vi "HeaterAlarmStatusChanged.vi"(7 "ControlQueue":refnum<queue>, 8 "error in (no error)":errorcluster, 9 "HeaterAlarmStatus":bool, 10 "HeaterAlarmStatusChanged":bool, 11 "DAQmxTaksContainer_General in":refnum<class "DAQmxTaksContainer_General.lvclass">) -> (0 "error out":errorcluster, 2 "Alarm":bool, 3 "DAQmxTaksContainer_General out":refnum<class "DAQmxTaksContainer_General.lvclass">)   [LabVIEW 2020, in "DAQmxTaksContainer_General.lvclass"]
uses:
  DAQmxTaksContainer_General.lvclass
  C:/dev/TRANCON/Classes/GeneralFunctionality/GeneralFunctionality.lvclass
  DAQmxTaksContainer_General.lvclass/DAQmxTaksContainer_General.ctl
  dependecies/ControlsVIs/Clusters-def/Standard Command.ctl
  dependecies/ControlsVIs/Clusters-def/SERVER-Commands.ctl
  dependecies/ControlsVIs/Clusters-def/ProtypeCommand-DAQmxReply.ctl
  dependecies/ControlsVIs/Clusters-def/Message types.ctl
  DAQmxTask.lvclass
  Control/Control-Server/Control-Server.lvclass
  Message/Message.lvclass
  GeneralFunctionality/GeneralFunctionality.lvclass
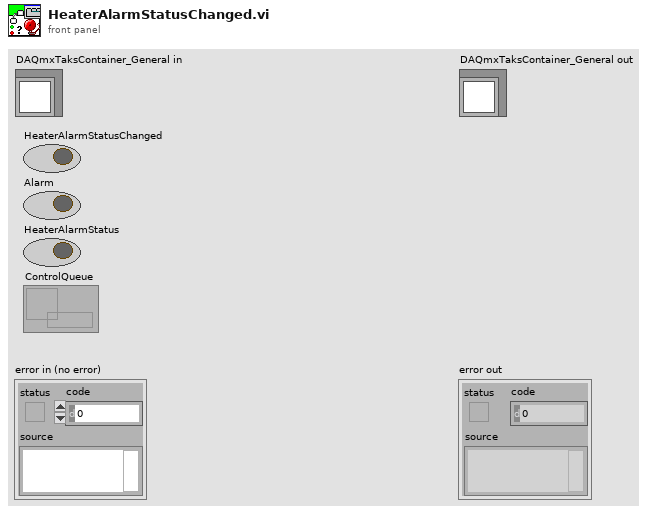
[diagram p1: front panel]
types:
  T1 = typedef "Message types.ctl" = string
  T2 = typedef "ProtypeCommand-DAQmxReply.ctl" = cluster{"On/Off":bool, "error out":errorcluster}
  T3 = typedef "Control-Server.lvclass/SERVER-Commands.ctl" = string
  T4 = typedef "Standard Command.ctl" = cluster{"command":string, "data":variant}
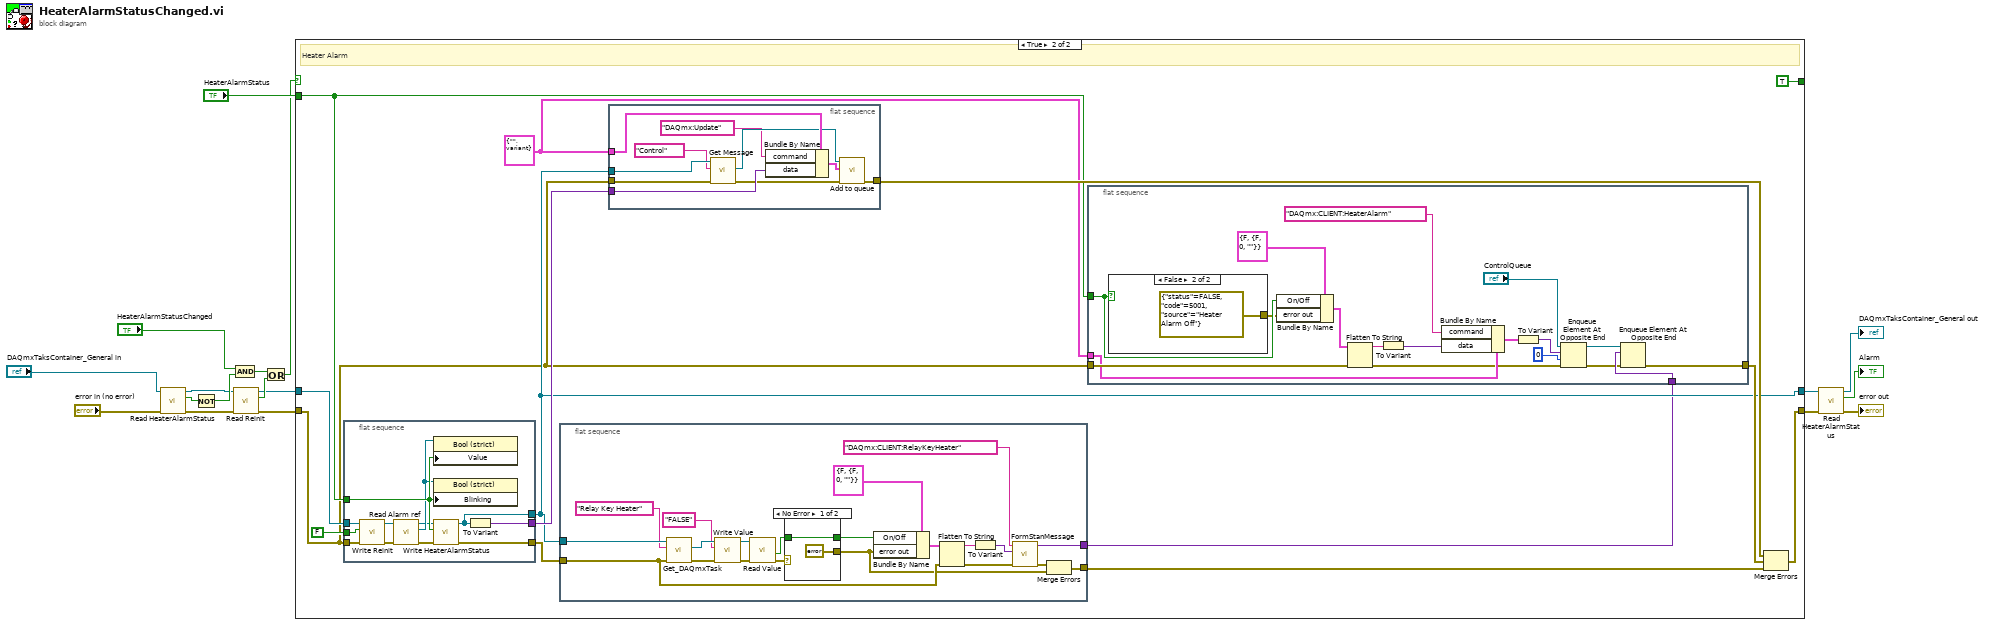
[diagram p0: block diagram]
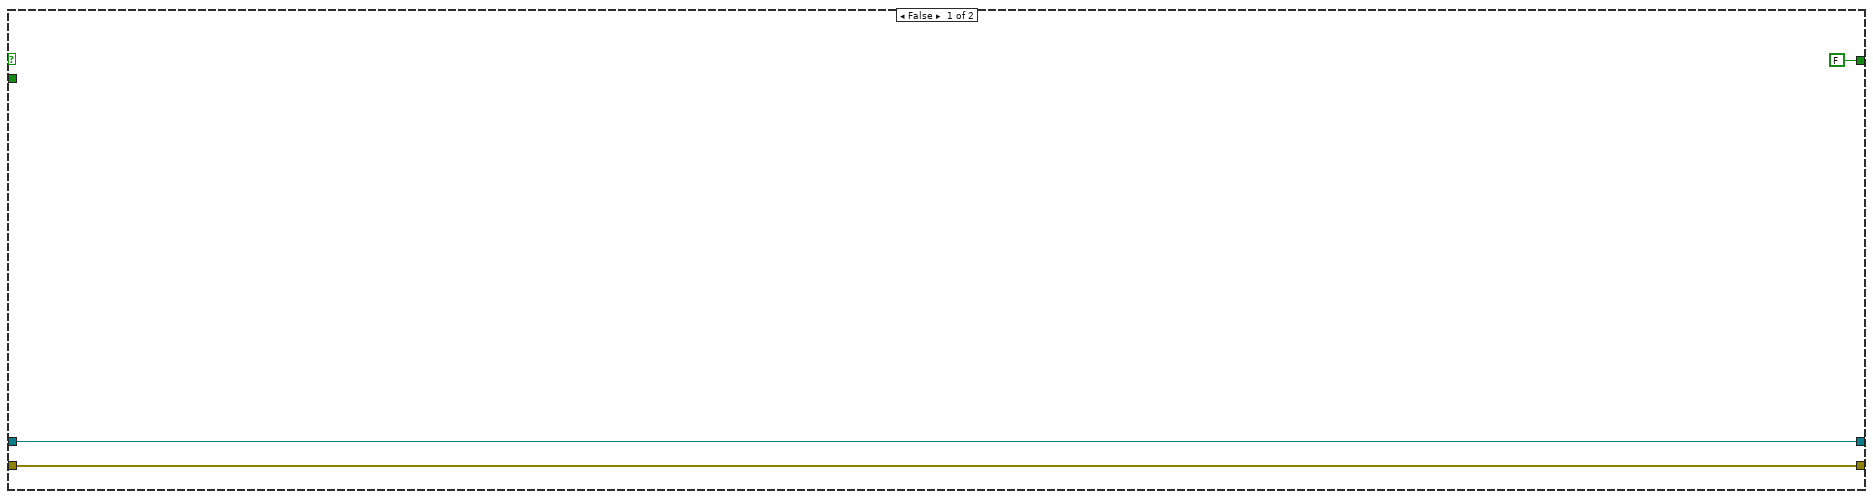
[diagram p2: hidden frame]
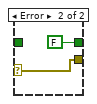
[diagram p3: hidden frame]
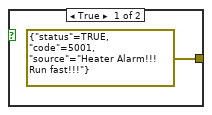
[diagram p4: hidden frame]
diagram:
  n1 = call "Read HeaterAlarmStatus.vi"("error in (no error)"="error in (no error)", "DAQmxTaksContainer_General in"="DAQmxTaksContainer_General in") -> ("error out"=w11:errorcluster, "HeaterAlarmStatus"=w13:bool, "DAQmxTaksContainer_General out"=w9:refnum<class "DAQmxTaksContainer_General.lvclass">)  [unwired: 7 in]
  n2 = Not(x=w13) -> (.not. x?=w16:bool)
  n3 = And(x="HeaterAlarmStatusChanged", y=w16) -> (x .and. y?=w15:bool)
  n4 = call "Read Reinit.vi"("error in (no error)"=w11, "DAQmxTaksContainer_General in"=w9) -> ("error out"=w10:errorcluster, "Reinit"=w12:bool, "DAQmxTaksContainer_General out"=w8:refnum<class "DAQmxTaksContainer_General.lvclass">)  [unwired: 7 in]
  n5 = Or(x=w15, y=w12) -> (x .or. y?=w14:bool)
  n6 = case shown="True" w14 {
    tunnel: [w21 w34] -> w7
    tunnel: [FALSE ("Alarm") TRUE ("Alarm")] -> _
    tunnel: w8 -> [w19 w25]
    tunnel: w10 -> [w21 w22]
    tunnel: [w19 w27] -> w5
    tunnel: "HeaterAlarmStatus" -> [_ w29]
    frame False {
    }
    frame True {
      w32 = T4 {"command"="", "data"=variant} ("input cluster")
      # "Heater Alarm"
      n7 = flat-sequence {
        tunnel: [w47] -> w31
        tunnel: w29 -> [w45]
        tunnel: [w46] -> w27
        tunnel: w25 -> [w38]
        tunnel: [w41] -> w24
        tunnel: FALSE ("AlarmOccured") -> [w40]
        tunnel: w22 -> [w36]
        frame #0 {
          n8 = call "Write Reinit.vi"("error in (no error)"=w36, "Reinit"=w40, "DAQmxTaksContainer_General in"=w38) -> ("error out"=w39:errorcluster, "DAQmxTaksContainer_General out"=w37:refnum<class "DAQmxTaksContainer_General.lvclass">)  [unwired: 7 in]
          n9 = call "Read Alarm ref.vi"("error in (no error)"=w39, "DAQmxTaksContainer_General in"=w37) -> ("error out"=w43:errorcluster, "Alarm"=w44:refnum<vi>, "DAQmxTaksContainer_General out"=w42:refnum<class "DAQmxTaksContainer_General.lvclass">)  [unwired: 7 in]
          n10 = property on="Property Node" class="Bool (strict)"(reference=w44, "Value"=w45) -> ()  [unwired: 1 in, 2 out]
          n11 = property on="Property Node" class="Bool (strict)"(reference=w44, "Blinking"=w45) -> ()  [unwired: 1 in, 2 out]
          n12 = call "Write HeaterAlarmStatus.vi"("error in (no error)"=w43, "HeaterAlarmStatus"=w45, "DAQmxTaksContainer_General in"=w42) -> ("error out"=w41:errorcluster, "DAQmxTaksContainer_General out"=w46:refnum<class "DAQmxTaksContainer_General.lvclass">)  [unwired: 7 in]
          n13 = To Variant(anything=w46) -> (Variant=w47:variant)
        }
      }
      n14 = flat-sequence {
        tunnel: w24 -> [w76]
        tunnel: w27 -> [w78]
        tunnel: [w75] -> w28
        tunnel: [w77] -> w26
        frame #0 {
          n15 = call "Get_DAQmxTask.vi"("error in (no error)"=w76, "Task name"="Relay Key Heater", "DAQmxTaksContainer_General in"=w78) -> ("error out"=w73:errorcluster, "DAQmx Task"=w74:refnum<class "DAQmxTask.lvclass">)  [unwired: 6 in, 1 out]
          n16 = call-dynamic "Write Value.vi"("error in (no error)"=w73, "Data"="FALSE", "DAQmxTask en entrée"=w74) -> ("error out"=w71:errorcluster, "DAQmxTask en sortie"=w70:refnum<class "DAQmxTask.lvclass">)  [unwired: 7 in]
          n17 = call-dynamic "Read Value.vi"("error in (no error)"=w71, "DAQmxTask en entrée"=w70) -> ("error out"=w63:errorcluster, "Data"=w62:bool)  [unwired: 6 in, 2 out]
          n18 = case shown="No Error" w63 {
            selector: w63 -> [_ w82]
            tunnel: [errorcluster {"status"=FALSE, "code"=5001, "source"="Relay key heater worked"} ("error constant") w82] -> w59
            tunnel: w62 -> [w79 _]
            tunnel: [w79 FALSE] -> w61
            frame No Error {
            }
            frame Error {
            }
          }
          n19 = Bundle By Name(cluster=T2 {"On/Off"=FALSE, "error out"={"status"=FALSE, "code"=0, "source"=""}} ("output cluster"), "On/Off"=w61, "error out"=w59) -> (w66:T2)
          n20 = Flatten To String(anything=w66, error in (no error)=w76) -> (data string=w65:string, error out=w69:errorcluster)  [unwired: 2 in, 1 out]
          n21 = To Variant(anything=w65) -> (Variant=w68:variant)
          n22 = call "FormStanMessage.vi"("error in"=w69, "data"=w68, "Command"=T3 "DAQmx:CLIENT:RelayKeyHeater" ("command")) -> ("error out"=w60:errorcluster, "message"=w77:variant)  [unwired: 7 in]
          n23 = Merge Errors(w60, w59) -> (w75:errorcluster)
        }
      }
      n24 = flat-sequence {
        tunnel: w22 -> [w57]
        tunnel: [w56] -> w33
        tunnel: w32 -> [w55]
        tunnel: w31 -> [w54]
        tunnel: w27 -> [w53]
        frame #0 {
          n25 = call "Get Message.vi"("error in (no error)"=w57, "Message type"=T1 "Control", "GeneralFunctionality en entrée"=w53) -> ("error out"=w51:errorcluster, "Message.lvclass"=w52:refnum<class "Message.lvclass">)  [unwired: 6 in, 1 out]
          n26 = Bundle By Name(cluster=w55, "command"="DAQmx:Update", "data"=w54) -> (w49:T4)
          n27 = call "Add to queue.vi"("error in (no error)"=w51, "Data"=w49, "Message in"=w52) -> ("error out"=w56:errorcluster)  [unwired: 7 in, 1 out]
        }
      }
      n28 = flat-sequence {
        tunnel: w22 -> [w100]
        tunnel: w32 -> [w99]
        tunnel: [w97] -> w30
        tunnel: w29 -> [w98]
        tunnel: w26 -> [w96]
        frame #0 {
          n29 = case shown="False" w98 {
            tunnel: [errorcluster {"status"=TRUE, "code"=5001, "source"="Heater Alarm!!! Run fast!!!"} ("error out") errorcluster {"status"=FALSE, "code"=5001, "source"="Heater Alarm Off"} ("error out")] -> w91
            frame True {
            }
            frame False {
            }
          }
          n30 = Bundle By Name(cluster=T2 {"On/Off"=FALSE, "error out"={"status"=FALSE, "code"=0, "source"=""}} ("output cluster"), "On/Off"=w98, "error out"=w91) -> (w92:T2)
          n31 = Flatten To String(anything=w92, error in (no error)=w100) -> (data string=w95:string, error out=w85:errorcluster)  [unwired: 2 in, 1 out]
          n32 = To Variant(anything=w95) -> (Variant=w94:variant)
          n33 = Bundle By Name(cluster=w99, "command"=T3 "DAQmx:CLIENT:HeaterAlarm" ("Command"), "data"=w94) -> (w93:T4)
          n34 = To Variant(anything=w93) -> (Variant=w88:variant)
          n35 = Enqueue Element At Opposite End(queue="ControlQueue", element=w88, timeout in ms (-1)=0 ("timeout en ms (-1)"), error in (no error)=w85) -> (queue out=w83:refnum<queue>, error out=w84:errorcluster)  [unwired: 1 out]
          n36 = Enqueue Element At Opposite End(queue=w83, element=w96, error in (no error)=w84) -> (error out=w97:errorcluster)  [unwired: 1 in, 2 out]
        }
      }
      n37 = Merge Errors(w33, w30, w28) -> (w34:errorcluster)
    }
  }
  n38 = call "Read HeaterAlarmStatus.vi"("error in (no error)"=w7, "DAQmxTaksContainer_General in"=w5) -> ("error out"=→"error out":errorcluster, "HeaterAlarmStatus"=→"Alarm":bool, "DAQmxTaksContainer_General out"=→"DAQmxTaksContainer_General out":refnum<class "DAQmxTaksContainer_General.lvclass">)  [unwired: 7 in]
